vi "afg_test.vi"() -> ()   [LabVIEW 2020]
uses:
  General AC source/Type definitions/AC Source.ctl
  General AC source/Type definitions/AC Source type.ctl
  0d06c1dc-2d6d-41c6-94dd-a16baf8240bb.vi
  <vilib>/Comparison/Less/Less Functor/Less Functor.lvclass
panel:
  in  "repetitions for one timeout":i32=10
  out "error out 3":errorcluster
  out "error out 2":errorcluster
  out "error out 1":errorcluster
  out "iteration":i32
  out "timeout (ms)":i32
  out "error in (no error)":errorcluster
  in  "AC source":T1={"AC Source type"=enum."Tektronix AFG3000 series", "VISA"="", "Ref. clock (Hz)"=10000000.0, "status ref"=refnum}
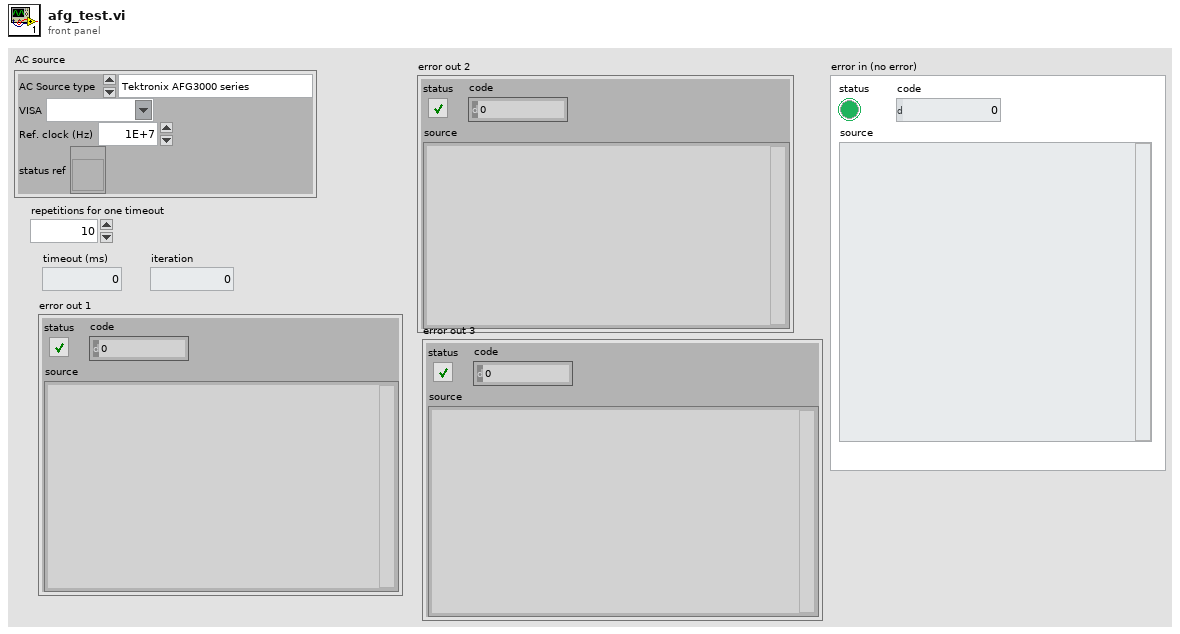
[diagram p1: front panel]
types:
  T1 = typedef "AC Source.ctl" = cluster{"AC Source type":T2, "VISA":refnum<visa-resource-name>, "Ref. clock (Hz)":dbl, "status ref":refnum<vi>}
  T2 = typedef "AC Source type.ctl" = enum16{"Fluke 5XXX calibrator", "Tektronix AFG3000 series", "dummy"}
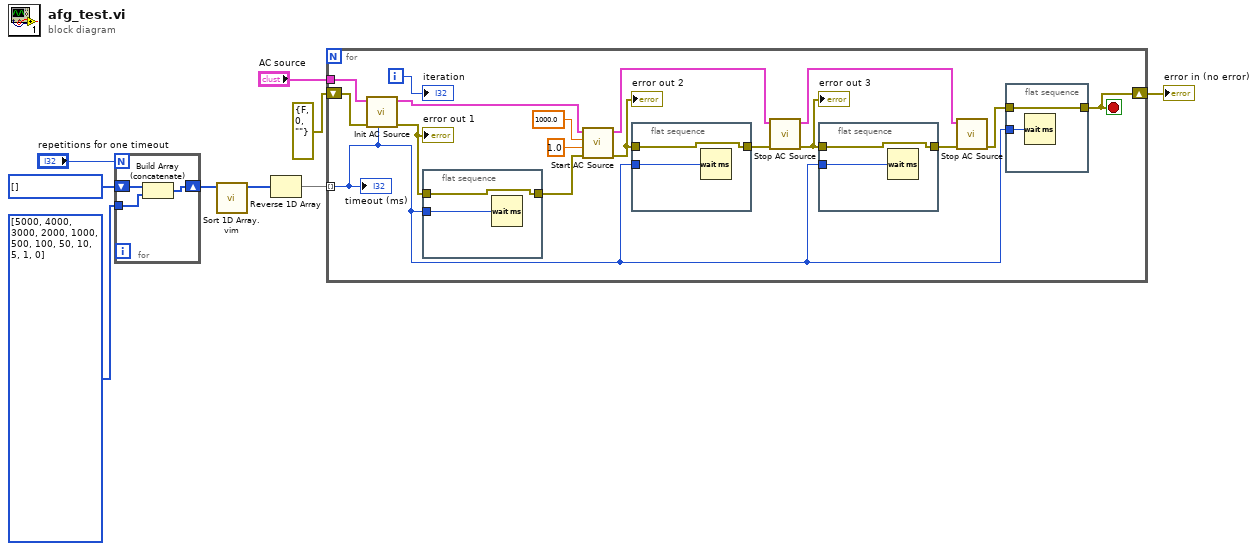
[diagram p0: block diagram]
diagram:
  n1 = for {
    N: "repetitions for one timeout" -> [_]
    shift-right: [w10] -> w2
    shift-left: i32[] [] -> [w11]
    tunnel: i32[] [5000, 4000, 3000, 2000, 1000, 500, 100, 50, 10, 5, 1, 0] -> [w12]
    n2 = Build Array (concatenate)(w11, w12) -> (w10:i32[])
  }
  n3 = call "Sort 1D Array.vim"("unsorted array"=w2) -> ("sorted array"=w6:i32[])  [unwired: 10 in]
  n4 = Reverse 1D Array(array=w6) -> (reversed array=w5:i32[])
  n5 = for {
    tunnel: "AC source" -> [w29]
    shift-right: [w15] -> w7
    shift-left: errorcluster {"status"=FALSE, "code"=0, "source"=""} ("error in (no error)") -> [w25]
    tunnel: w5 -> [w13] mode=indexing
    i -> [w24]
    stop <- w15 stop-if-true
    n6 = call "Init AC Source.vi"("General Settings:Timeout Value"=w13, "error in (no error)"=w25, "AC source"=w29) -> ("error out"=w21:errorcluster, "AC source out"=w28:T1)  [unwired: 6 in, 1 out]
    "error out 1" <- w21
    n7 = flat-sequence {
      tunnel: w13 -> [w37]
      tunnel: w21 -> [w36]
      tunnel: [w36] -> w20
      frame #0 {
        n8 = Wait (ms)(milliseconds to wait=w37) -> ()  [unwired: 1 out]
      }
    }
    n9 = call "Start AC Source.vi"("error in (no error)"=w20, "Signal amplitude (V)"=1.0, "Signal frequency  (Hz)"=1000.0, "AC source"=w28) -> ("error out"=w18:errorcluster, "AC source out"=w27:T1)  [unwired: 5 in, 1 out]
    "error out 2" <- w18
    n10 = flat-sequence {
      tunnel: w13 -> [w35]
      tunnel: [w34] -> w19
      tunnel: w18 -> [w34]
      frame #0 {
        n11 = Wait (ms)(milliseconds to wait=w35) -> ()  [unwired: 1 out]
      }
    }
    n12 = call "Stop AC Source.vi"("error in (no error)"=w19, "AC source"=w27) -> ("error out"=w16:errorcluster, "AC source out"=w26:T1)  [unwired: 8 in]
    "error out 3" <- w16
    n13 = flat-sequence {
      tunnel: w13 -> [w33]
      tunnel: [w32] -> w17
      tunnel: w16 -> [w32]
      frame #0 {
        n14 = Wait (ms)(milliseconds to wait=w33) -> ()  [unwired: 1 out]
      }
    }
    n15 = call "Stop AC Source.vi"("error in (no error)"=w17, "AC source"=w26) -> ("error out"=w14:errorcluster)  [unwired: 8 in, 1 out]
    n16 = flat-sequence {
      tunnel: w13 -> [w31]
      tunnel: [w30] -> w15
      tunnel: w14 -> [w30]
      frame #0 {
        n17 = Wait (ms)(milliseconds to wait=w31) -> ()  [unwired: 1 out]
      }
    }
    "timeout (ms)" <- w13
    "iteration" <- w24
  }
  "error in (no error)" <- w7
